vi "Set to mouse position.vi"(7 "Open at mouse position?":bool, 8 "error in (no error)":errorcluster, 11 "Window position to set":T1) -> (0 "error out":errorcluster, 3 "New window position to set":T1)   [LabVIEW 2020]
uses:
  <vilib>/Utility/miscctls.llb/LVRectTypeDef.ctl
panel:
  out "Y size":i16
  out "X-size":i16
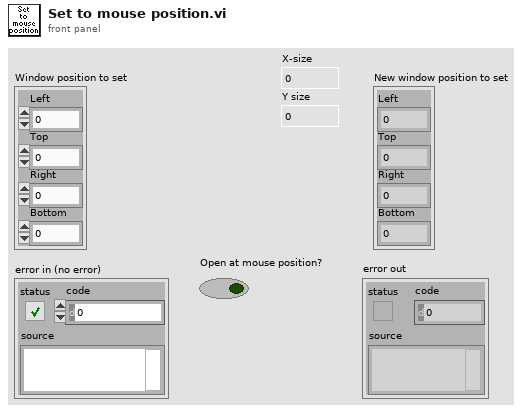
[diagram p1: front panel]
types:
  T1 = typedef "LVRectTypeDef.ctl" = cluster{"Left":i16, "Top":i16, "Right":i16, "Bottom":i16}
  T2 = cluster{"Horizontal":i32, "Vertical":i32, "Scrolling":i32}
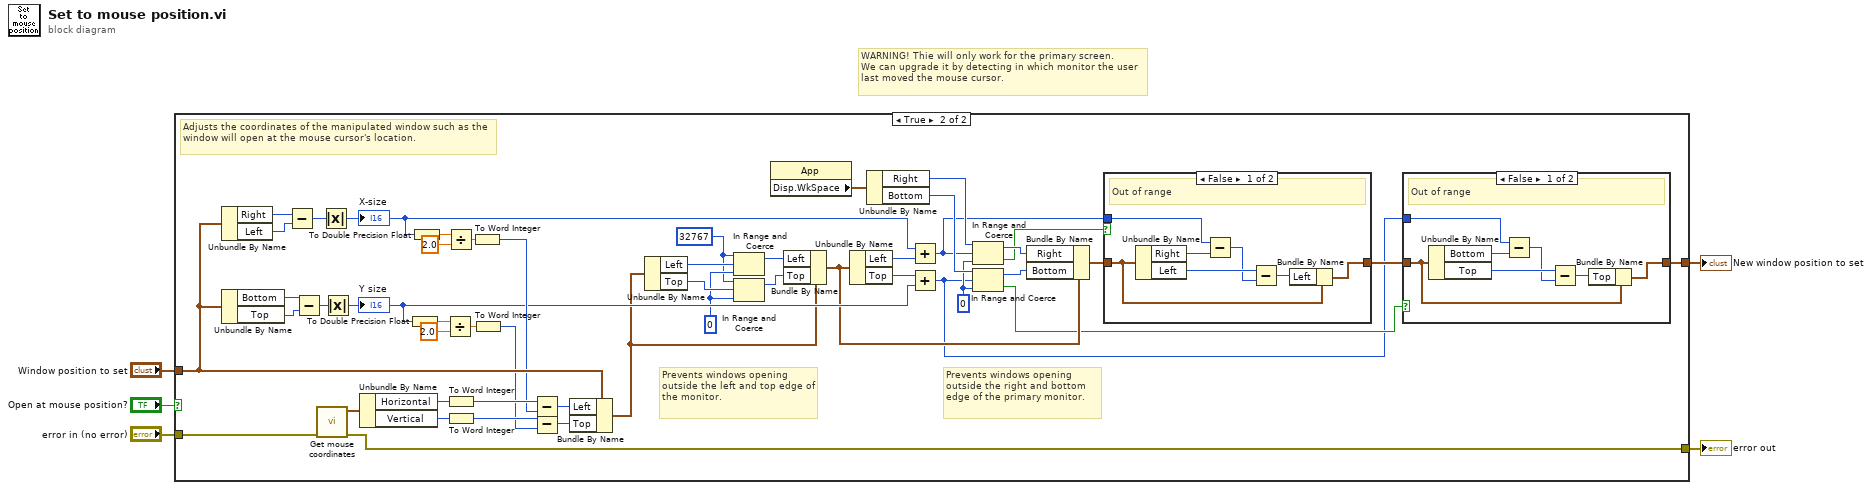
[diagram p0: block diagram]
diagram:
  # "WARNING! Thie will only work for the primary screen.\nWe can upgrade it by detecting in which monitor the user last moved the mouse cursor."
  n1 = case shown="True" "Open at mouse position?" {
    tunnel: "error in (no error)" -> [w6 w56]
    tunnel: [w6 w55] -> w4
    tunnel: "Window position to set" -> [w7 w53]
    tunnel: [w7 w8] -> w1
    frame False {
    }
    frame True {
      w14 = i16 0 ("lower limit")
      w27 = i16 32767 ("upper limit")
      w28 = i16 0 ("lower limit")
      # "Prevents windows opening outside the right and bottom edge of the primary monitor."
      # "Adjusts the coordinates of the manipulated window such as the window will open at the mouse cursor's location."
      # "Prevents windows opening outside the left and top edge of the monitor."
      n2 = Unbundle By Name(w53) -> ("Right"=w52:i16, "Left"=w51:i16)
      n3 = Unbundle By Name(w53) -> ("Bottom"=w49:i16, "Top"=w48:i16)
      n4 = Subtract(x=w52, y=w51) -> (x-y=w50:i16)
      n5 = Subtract(x=w49, y=w48) -> (x-y=w47:i16)
      n6 = call "Get mouse coordinates.vi"("error in"=w56) -> ("error out"=w55:errorcluster, "axis info"=w54:T2)  [unwired: 9 in]
      n7 = Absolute Value(x=w50) -> (abs(x)=w31:i16)
      "X-size" <- w31
      n8 = Absolute Value(x=w47) -> (abs(x)=w32:i16)
      "Y size" <- w32
      n9 = Unbundle By Name(w54) -> ("Horizontal"=w46:i32, "Vertical"=w45:i32)
      n10 = To Double Precision Float(number=w32) -> (double precision float=w42:dbl)
      n11 = To Double Precision Float(number=w31) -> (double precision float=w43:dbl)
      n12 = Divide(x=w42, y=2.0) -> (x/y=w40:dbl)
      n13 = Divide(x=w43, y=2.0) -> (x/y=w39:dbl)
      n14 = To Word Integer(number=w46) -> (16bit integer=w38:i16)
      n15 = To Word Integer(number=w45) -> (16bit integer=w35:i16)
      n16 = To Word Integer(number=w39) -> (16bit integer=w36:i16)
      n17 = To Word Integer(number=w40) -> (16bit integer=w34:i16)
      n18 = Subtract(x=w38, y=w36) -> (x-y=w37:i16)
      n19 = Subtract(x=w35, y=w34) -> (x-y=w33:i16)
      n20 = Bundle By Name(cluster=w53, "Left"=w37, "Top"=w33) -> (w22:T1)
      n21 = Unbundle By Name(w22) -> ("Left"=w30:i16, "Top"=w29:i16)
      n22 = In Range and Coerce(upper limit=w27, x=w30, lower limit=w28) -> (coerced(x)=w26:i16)  [unwired: 1 out]
      n23 = In Range and Coerce(upper limit=w27, x=w29, lower limit=w28) -> (coerced(x)=w25:i16)  [unwired: 1 out]
      n24 = property class="App"() -> ("Disp.WkSpace"=w19:T1)  [unwired: 2 in, 2 out]
      n25 = Bundle By Name(cluster=w22, "Left"=w26, "Top"=w25) -> (w21:T1)
      n26 = Unbundle By Name(w21) -> ("Left"=w24:i16, "Top"=w23:i16)
      n27 = Unbundle By Name(w19) -> ("Right"=w16:i16, "Bottom"=w15:i16)
      n28 = Add(x=w31, y=w24) -> (x+y=w12:i16)
      n29 = Add(x=w23, y=w32) -> (x+y=w9:i16)
      n30 = In Range and Coerce(upper limit=w16, x=w12, lower limit=w14) -> (coerced(x)=w18:i16, In Range?=w13:bool)
      n31 = In Range and Coerce(upper limit=w15, x=w9, lower limit=w14) -> (coerced(x)=w17:i16, In Range?=w10:bool)
      n32 = Bundle By Name(cluster=w21, "Right"=w18, "Bottom"=w17) -> (w20:T1)
      n33 = case shown="False" w13 {
        tunnel: w20 -> [w69 w72]
        tunnel: [w65 w72] -> w11
        tunnel: w12 -> [w70 _]
        frame False {
          # "Out of range"
          n34 = Unbundle By Name(w69) -> ("Right"=w71:i16, "Left"=w68:i16)
          n35 = Subtract(x=w70, y=w71) -> (x-y=w66:i16)
          n36 = Subtract(x=w68, y=w66) -> (x-y=w67:i16)
          n37 = Bundle By Name(cluster=w69, "Left"=w67) -> (w65:T1)
        }
        frame True {
          # "In range"
        }
      }
      n38 = case shown="False" w10 {
        tunnel: w11 -> [w61 w64]
        tunnel: [w57 w64] -> w8
        tunnel: w9 -> [w62 _]
        frame False {
          # "Out of range"
          n39 = Unbundle By Name(w61) -> ("Bottom"=w63:i16, "Top"=w60:i16)
          n40 = Subtract(x=w62, y=w63) -> (x-y=w58:i16)
          n41 = Subtract(x=w60, y=w58) -> (x-y=w59:i16)
          n42 = Bundle By Name(cluster=w61, "Top"=w59) -> (w57:T1)
        }
        frame True {
          # "In range"
        }
      }
    }
  }
  "New window position to set" <- w1
  "error out" <- w4
